vi "Example_Port Code_cRIO.vi"(10 "Port":u8, 11 "FPGA I/O":T1={"SCLK"="DIO15", "CS_1"="DIO13", "MOSI"="DIO14", "MISO"="DIO12", "CS_2"="DIO11"}) -> ()   [LabVIEW 2011]
uses:
  Controls/FPGA SPI_Port Loop State.ctl
  <vilib>/rvi/DataTransferAndStorage/Container/Common/niFpgaContainerState.ctl
  <vilib>/rvi/DataTransferAndStorage/Container/Common/niFpgaDataTypeControl.ctl
  <vilib>/rvi/DataTransferAndStorage/Container/Common/niFpgaContainerImplementationControl.ctl
  <vilib>/rvi/DataTransferAndStorage/Container/Common/niFpgaContainerArbitrationOptionsControl.ctl
  <vilib>/rvi/DataTransferAndStorage/Container/Common/niFpgaTransferTypeControl.ctl
  <vilib>/rvi/DataTransferAndStorage/Container/Common/niFpgaContainerInitializationParameters.ctl
  <vilib>/rvi/Memory/Memory_Types/niFpgaMemoryInterfaceConfiguration.ctl
  <vilib>/rvi/FIFO/Fifo_Types/niFpgaFifoControlLogicControl.ctl
  <vilib>/rvi/DataTransferAndStorage/Container/Common/niFpgaContainerMetaDataKey.ctl
  Controls/FPGA SPI_SPI Loop State.ctl
  <vilib>/Platform/TimedLoop/XDataNode/timing_clust.ctl
  <vilib>/Platform/TimedLoop/XDataNode/nitl_modes.ctl
  <vilib>/Platform/TimedLoop/XDataNode/wakeup.ctl
  <vilib>/rvi/DataTransferAndStorage/Container/Common/niFpgaContainerGetUniqueNameForEmu.vi
  <vilib>/rvi/DataTransferAndStorage/Container/Common/niFpgaContainerSetEmuInfo.vi
  <vilib>/rvi/eio/common/nirviEmuReportErrorAndStop.vi
  Code/FPGA SPI_Globals.vi
  <vilib>/rvi/FIFO/Fifo_Resource/nirvififoEmulationSetSize.vi
  <vilib>/rvi/eio/common/nirviEmuTemplateMethod_errors.vi
  <vilib>/rvi/LocalResourceManager/LocalResourceManager.xnode
  <vilib>/Platform/TimedLoop/XDataNode/XDataNode.xnode
  <vilib>/rvi/DataTransferAndStorage/Container/XNode/niFpgaContainer.xnode
  <vilib>/rvi/FIFO/Fifo_Resource/nirvififoEmulationRead.vi
  <vilib>/rvi/FIFO/Fifo_Resource/nirvififoEmulationWrite.vi
  <vilib>/eio/EIONode/EIONode.xnode
  <vilib>/Platform/TimedLoop/XDataNode/XDNodeRunTimeDep.lvlib
panel:
  # "12 and 11 are NC"
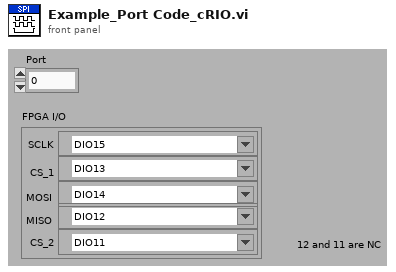
[diagram p1: front panel]
types:
  T1 = cluster{"SCLK":refnum<k21>, "CS_1":refnum<k21>, "MOSI":refnum<k21>, "MISO":refnum<k21>, "CS_2":refnum<k21>}
  T2 = cluster{"CS":u8, "CS Active State":bool, "CPOL":bool, "CPHA":bool, "Wait Ticks":u32}
  T3 = typedef "FPGA SPI_Port Loop State.ctl" = enum8{"Idle", "Start", "Configure Hardware", "Start Hardware", "Set Done", "Wait Until Done"}
  T4 = typedef "FPGA SPI_SPI Loop State.ctl" = enum8{"Initialize", "Read From FIFO", "Set CS", "Wait Before Set", "Set Clock", "Wait Before Reset", "Reset Clock", "Write to FIFO", "Reset CS"}
  T5 = typedef "XDNodeRunTimeDep.lvlib/timing_clust.ctl" = cluster{"Expected End [f-1]":u64, "Actual End [f-1]":u64, "Finished Late? [f-1]":bool, "Expected End [i-1]":u64, "Actual End [i-1]":u64, "Finished Late? [i-1]":bool, "Expected Start [i]":u64, "Actual Start [i]":u64, "Expected Start [f]":u64, "Actual Start [f]":u64, "Source Name":string, "Structure Name":string, "Period":i64, "Deadline":i64, "Offset":i64, "Start":i64, "Priority":i32, "Timeout":i32, "Mode":T6, "Wakeup Reason":T7, "Error":errorcluster, "Source Type":string, "Secondary Source Type":string, "Global End Time":u64, "Global Start Time":u64, "Frame Duration":u64, "Iteration Duration":u64, "Assigned CPU":i32, "I/O Scan Engine Mode":u32}
  T6 = typedef "XDNodeRunTimeDep.lvlib/nitl_modes.ctl" = enum32{"No Change", "Process missed periods, maintain original phase", "Discard missed periods, maintain original phase", "Process missed periods, ignore original phase", "Discard missed periods, ignore original phase"}
  T7 = typedef "XDNodeRunTimeDep.lvlib/wakeup.ctl" = enum32{"Normal", "Aborted", "Asynchronous wakeup", "Timing source error", "Timed loop error", "Timeout"}
  T8 = typedef "FPGA SPI_Cmd.ctl" = enum8{"Idle", "Write/Read SPI", "Configure"}
  T9 = cluster{"MOSI":bool[], "MISO":bool[], "MOSI Byte Index":i8, "MISO Byte Index":i8}
  T10 = cluster{"Next State":T4, "Wait Count":u32, "Total Bits":u16, "Current Bit":u16, "Total Bytes":u16}
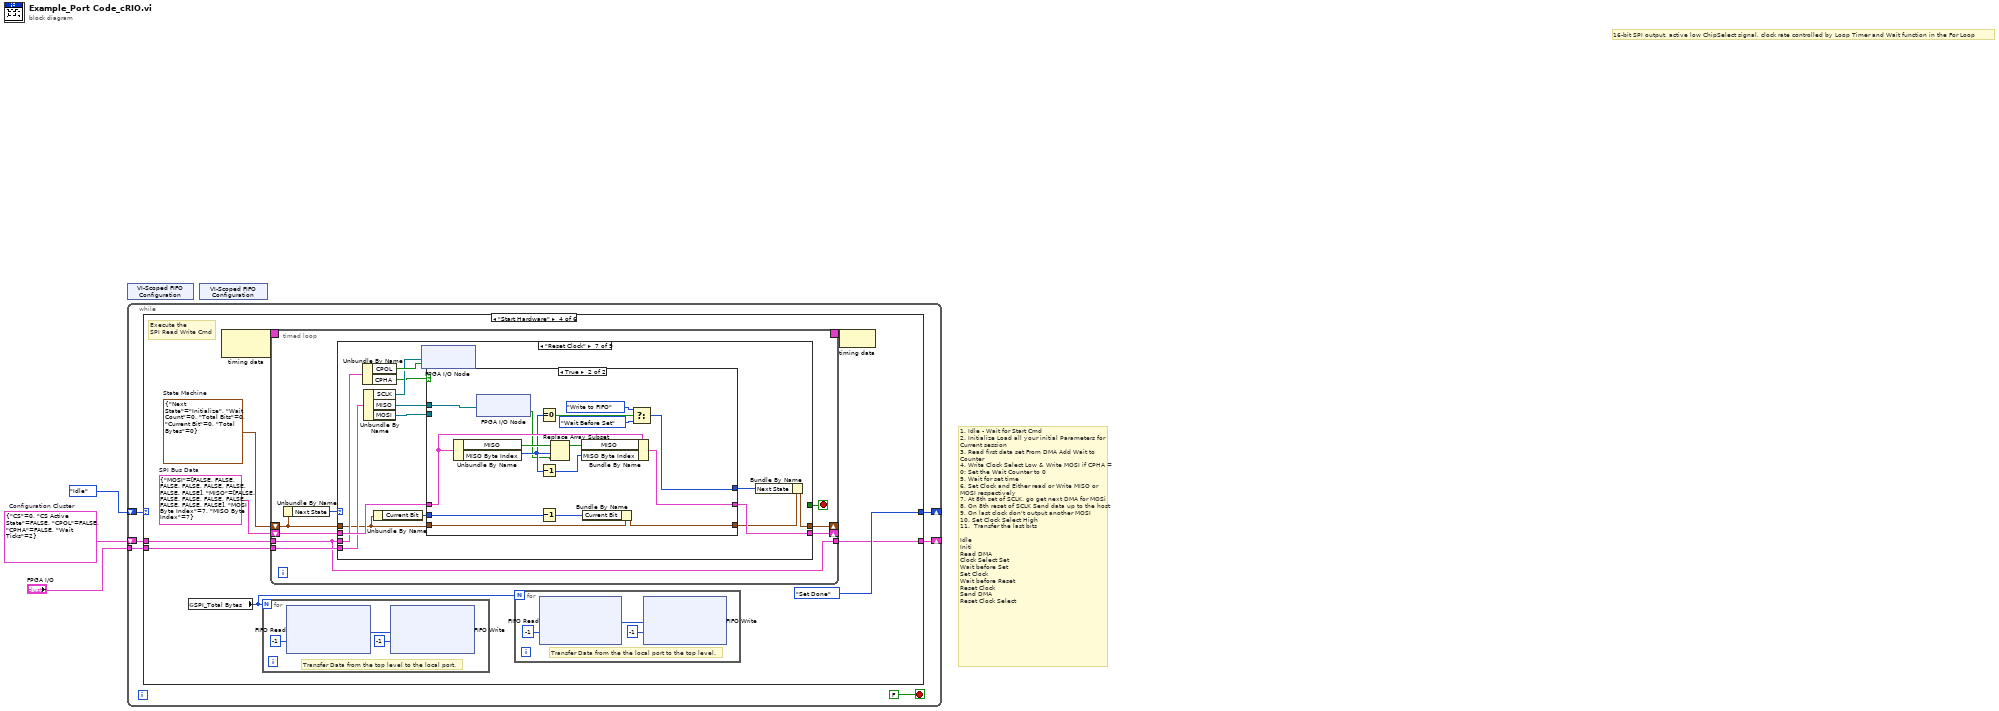
[diagram p0: block diagram]
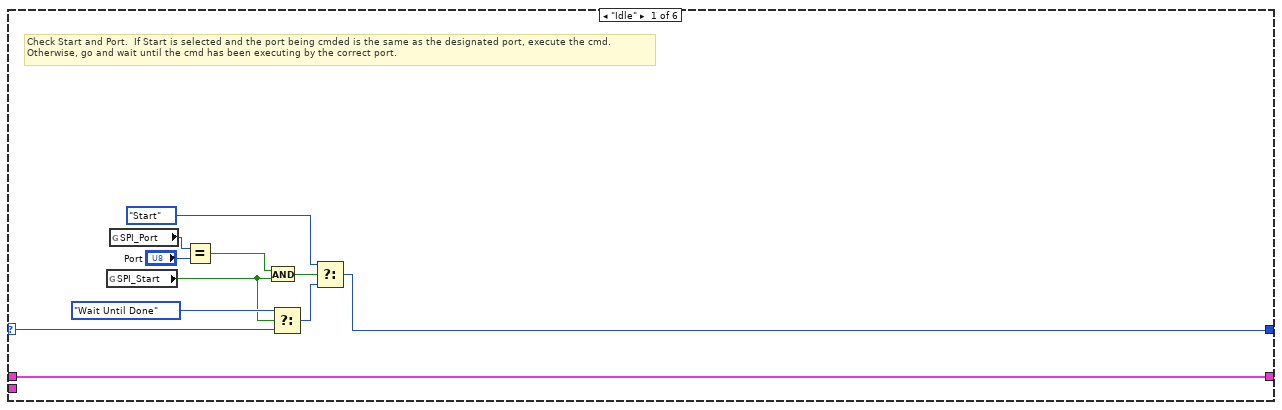
[diagram p2: hidden frame]
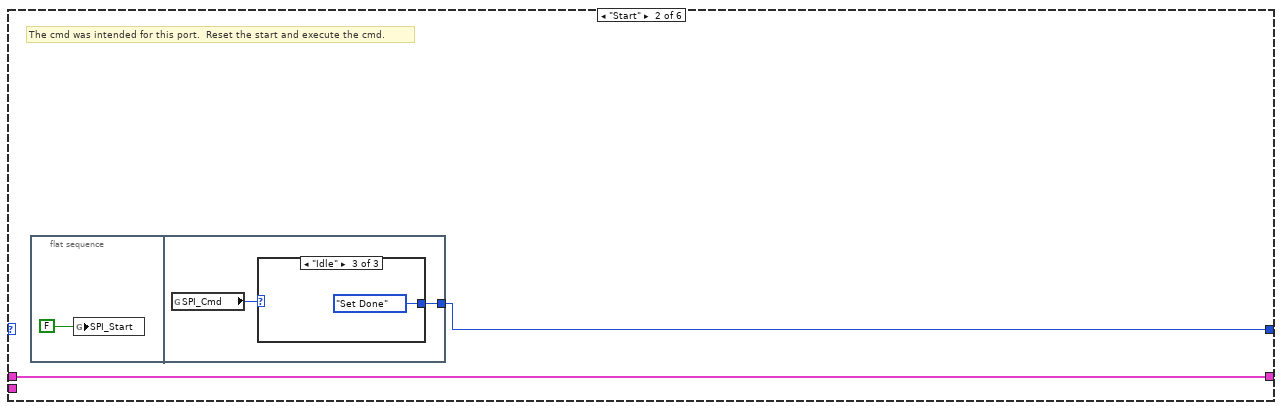
[diagram p3: hidden frame]
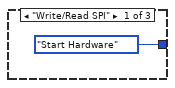
[diagram p4: hidden frame]
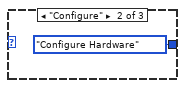
[diagram p5: hidden frame]
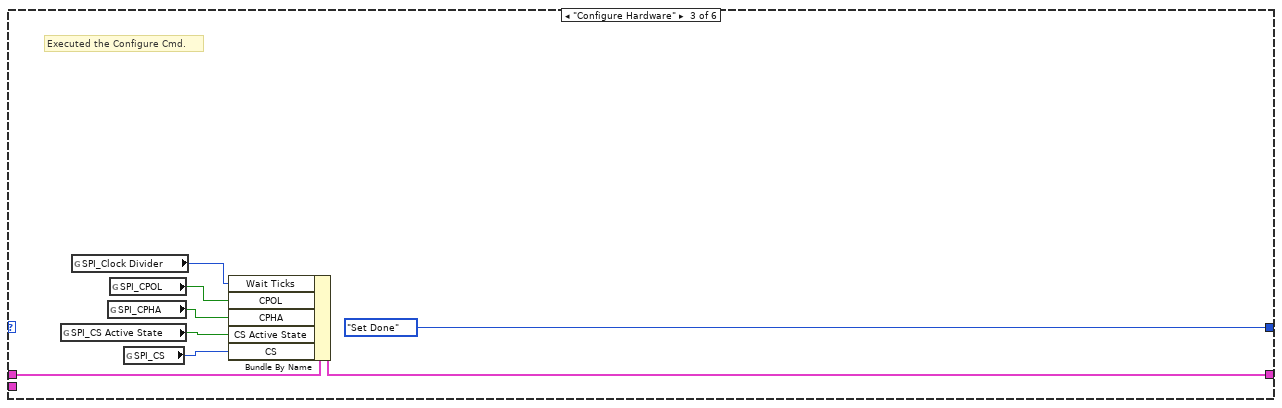
[diagram p6: hidden frame]
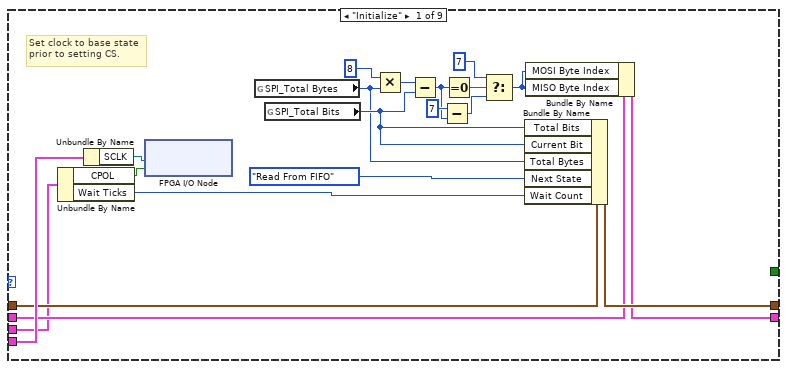
[diagram p7: hidden frame]
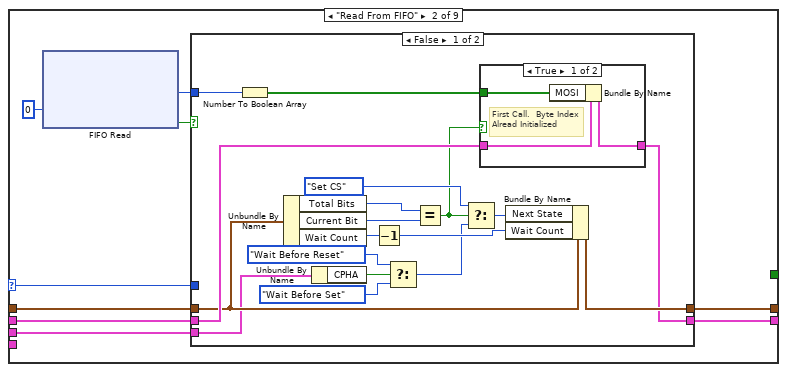
[diagram p8: hidden frame]
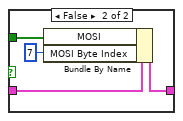
[diagram p9: hidden frame]
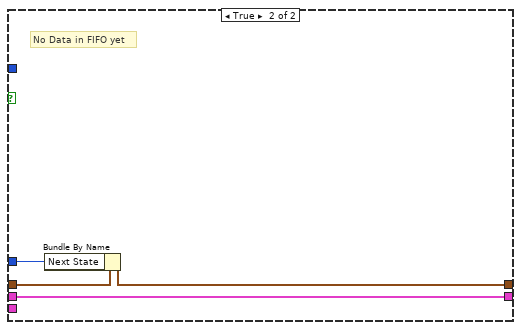
[diagram p10: hidden frame]
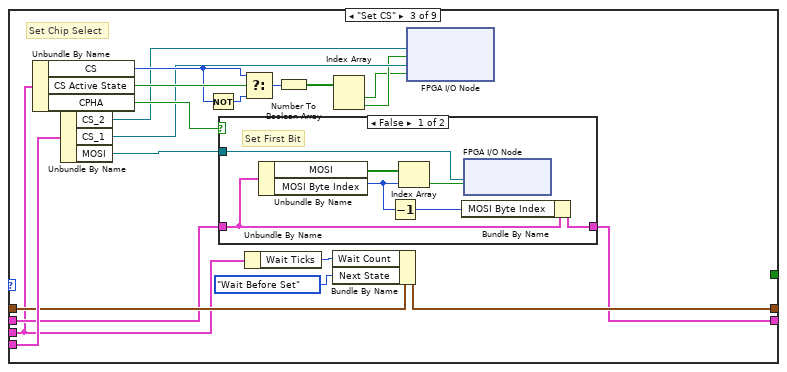
[diagram p11: hidden frame]
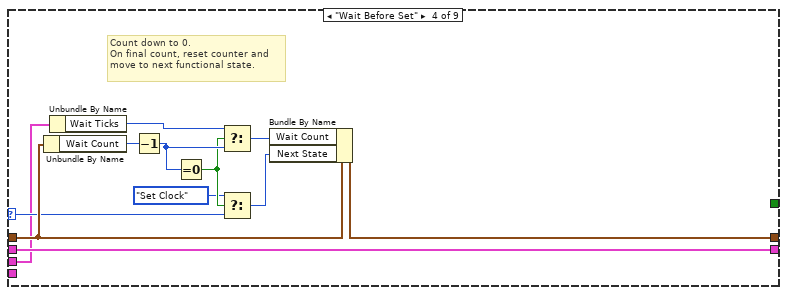
[diagram p13: hidden frame]
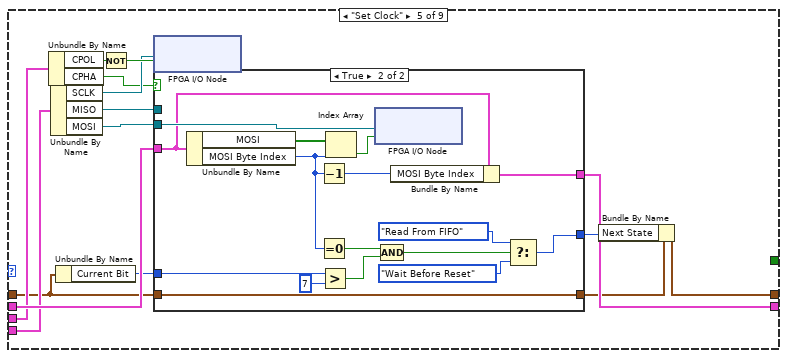
[diagram p14: hidden frame]
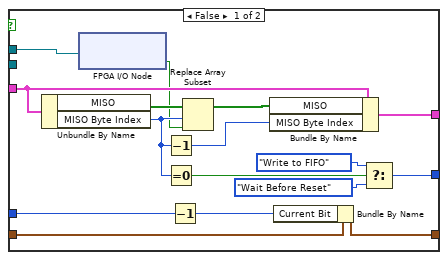
[diagram p15: hidden frame]
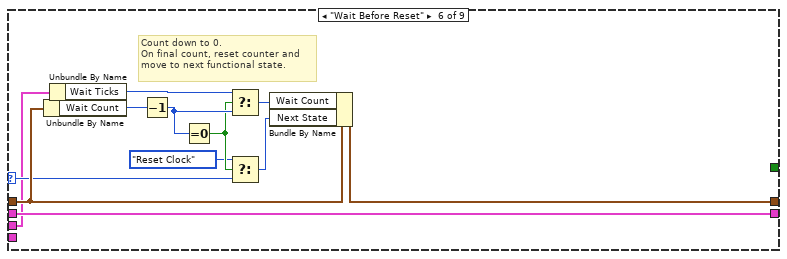
[diagram p16: hidden frame]
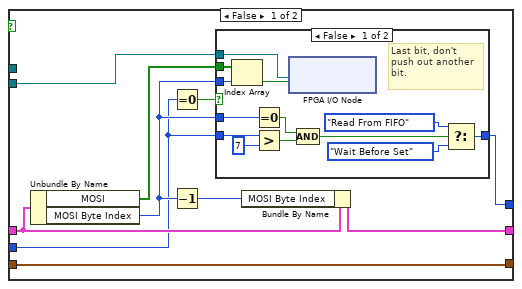
[diagram p17: hidden frame]
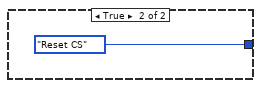
[diagram p18: hidden frame]
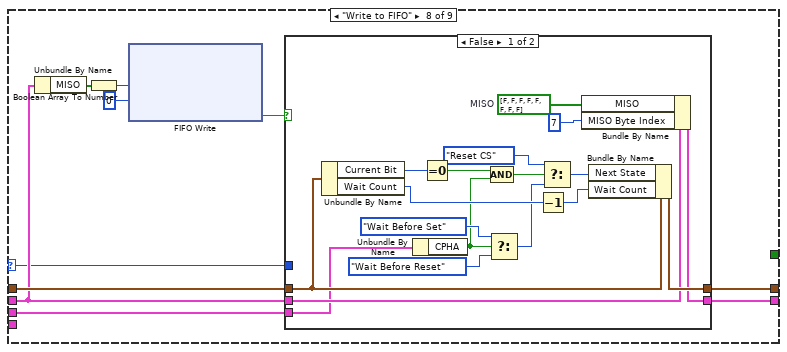
[diagram p19: hidden frame]
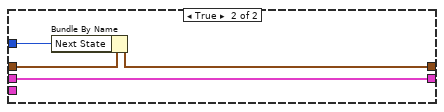
[diagram p20: hidden frame]
diagram:
  w2 = T2 {"CS"=0, "CS Active State"=FALSE, "CPOL"=FALSE, "CPHA"=FALSE, "Wait Ticks"=2}  # Configuration Cluster
  # "16-bit SPI output, active low ChipSelect signal, clock rate controlled by Loop Timer and Wait function in the For Loop"
  # "1. Idle - Wait for Start Cmd\n2. Initialize Load all your initial Parameters for Current session\n3. Read first data set From DMA Add Wait to Counter\n4. Write Clock Select Low & Write MOSI if CPHA = 0; Set the Wait Counter to 0\n5. Wait for set time\n6. Set Clock and Either read or Write MISO or MOSI respectively\n7. At 8th set of SCLK, go get next DMA for MOSi\n8. On 8th reset of SCLK Send data up to the host\n9. On last clock don't output another MOSI\n10. Set Clock Select High \n11.  Transfer the last bits\n\nIdle\nIniti\nRead DMA\nClock Select Set\nWait before Set\nSet Clock\nWait before Reset\nReset Clock\nSend DMA\nReset Clock Select"
  n1 = xnode "VI-Scoped FIFO Configuration"() -> ()  [unwired: 1 out]
  n2 = while {
    shift-right: [w8] -> _
    shift-left: FPGA_SPI_Port_Loop_State."Idle" ("Action") -> [w7]
    shift-right: [w4] -> _
    shift-left: w2 -> [w6]
    tunnel: "FPGA I/O" -> [w5]
    stop <- FALSE stop-if-true
    n3 = case shown="\"Start Hardware\"" w7 {
      selector: w7 -> [w10 _ _ _ _ w322]
      tunnel: [w19 w22 FPGA_SPI_Port_Loop_State."Set Done" ("Action") FPGA_SPI_Port_Loop_State."Set Done" ("Action") FPGA_SPI_Port_Loop_State."Idle" ("Action") w321] -> w8
      tunnel: w6 -> [w14 w21 w32 w37 w317 w320]
      tunnel: w5 -> [_ _ _ w42 _ _]
      tunnel: [w14 w21 w31 w38 w317 w320] -> w4
      frame "Idle" {
        # "Check Start and Port.  If Start is selected and the port being cmded is the same as the designated port, execute the cmd.\nOtherwise, go and wait until the cmd has been executing by the correct port."
        n4 = global read "FPGA SPI_Globals.vi" "SPI_Start"() -> (w11:bool)
        n5 = global read "FPGA SPI_Globals.vi" "SPI_Port"() -> (w18:u8)
        n6 = Equal?(x=w18, y="Port") -> (x = y?=w12:bool)
        n7 = And(x=w12, y=w11) -> (x .and. y?=w16:bool)
        n8 = Select(t=FPGA_SPI_Port_Loop_State."Wait Until Done" ("Action"), s=w11, f=w10) -> (s? t:f=w15:T3)
        n9 = Select(t=FPGA_SPI_Port_Loop_State."Start" ("Action"), s=w16, f=w15) -> (s? t:f=w19:T3)
      }
      frame "Start" {
        # "The cmd was intended for this port.  Reset the start and execute the cmd."
        n10 = flat-sequence {
          tunnel: [w24] -> w22
          frame #0 {
            n11 = global write "FPGA SPI_Globals.vi" "SPI_Start"(FALSE ("Write Flag")) -> ()
          }
          frame #1 {
            n12 = global read "FPGA SPI_Globals.vi" "SPI_Cmd"() -> (w25:T8)
            n13 = case shown="\"Idle\"" w25 {
              tunnel: [FPGA_SPI_Port_Loop_State."Start Hardware" ("Action") FPGA_SPI_Port_Loop_State."Configure Hardware" ("Action") FPGA_SPI_Port_Loop_State."Set Done" ("Action")] -> w24
              frame "Write/Read SPI" {
              }
              frame "Configure" {
              }
              frame "Idle" {
              }
            }
          }
        }
      }
      frame "Configure Hardware" {
        # "Executed the Configure Cmd."
        n14 = global read "FPGA SPI_Globals.vi" "SPI_CS Active State"() -> (w34:bool)
        n15 = global read "FPGA SPI_Globals.vi" "SPI_Clock Divider"() -> (w29:u32)
        n16 = global read "FPGA SPI_Globals.vi" "SPI_CPHA"() -> (w33:bool)
        n17 = global read "FPGA SPI_Globals.vi" "SPI_CPOL"() -> (w36:bool)
        n18 = global read "FPGA SPI_Globals.vi" "SPI_CS"() -> (w35:u8)
        n19 = Bundle By Name(cluster=w32, "Wait Ticks"=w29, "CPOL"=w36, "CPHA"=w33, "CS Active State"=w34, "CS"=w35) -> (w31:T2)
      }
      frame "Start Hardware" {
        w40 = T9 {"MOSI"=[FALSE, FALSE, FALSE, FALSE, FALSE, FALSE, FALSE, FALSE], "MISO"=[FALSE, FALSE, FALSE, FALSE, FALSE, FALSE, FALSE, FALSE], "MOSI Byte Index"=7, "MISO Byte Index"=7}  # SPI Bus Data
        w41 = T10 {"Next State"=enum."Initialize", "Wait Count"=0, "Total Bits"=0, "Current Bit"=0, "Total Bytes"=0}  # State Machine
        # "Execute the \nSPI Read Write Cmd"
        n20 = global read "FPGA SPI_Globals.vi" "SPI_Total Bytes"() -> (w39:u16)
        n21 = node-c288() -> (w44:T5)  [unwired: 1 out]
        n22 = for {
          N: w39 -> [_]
          # "Transfer Data from the top level to the local port."
          n23 = xnode ("FIFO Read")("Timeout"=-1) -> ("Element"=w50:u8)  [unwired: 1 in, 2 out]
          n24 = xnode ("FIFO Write")("Element"=w50, "Timeout"=-1) -> ()  [unwired: 1 in, 2 out]
        }
        n25 = timed-loop {
          timing-out: [_] -> w43
          timing: w44 -> [_]
          shift-right: [w59] -> _
          shift-left: w41 -> [w58]
          shift-right: [w55] -> _
          shift-left: w40 -> [w56]
          tunnel: w42 -> [w53]
          tunnel: [w52] -> w38
          tunnel: w37 -> [w52]
          stop <- w54 stop-if-true
          n26 = Unbundle By Name(w58) -> ("Next State"=w57:T4)
          n27 = case shown="\"Reset Clock\"" w57 {
            selector: w57 -> [_ w80 _ w149 _ w207 _ w270 _]
            tunnel: w58 -> [w76 w83 w129 w155 w159 w214 w217 w276 w311]
            tunnel: [w75 w86 w136 w156 w171 w215 w229 w277 w312] -> w59
            tunnel: w52 -> [w61 w82 w124 w146 w166 w205 w225 w274 w308]
            tunnel: w56 -> [w62 w84 w126 w147 w167 w212 w227 w273 w309]
            tunnel: [w65 w85 w125 w147 w168 w212 w226 w272 w309] -> w55
            tunnel: w53 -> [w79 _ w133 _ w165 _ w224 _ w306]
            tunnel: [_ _ _ _ _ _ _ _ TRUE ("Start Hardware")] -> w54
            frame "Initialize" {
              # "Set clock to base state\nprior to setting CS."
              n28 = Unbundle By Name(w61) -> ("CPOL"=w77:bool, "Wait Ticks"=w60:u32)
              n29 = Unbundle By Name(w79) -> ("SCLK"=w78:refnum<k21>)
              n30 = xnode "FPGA I/O Node"("I/O Item"=w77, "FPGA I/O In"=w78) -> ()  [unwired: 1 out]
              n31 = global read "FPGA SPI_Globals.vi" "SPI_Total Bytes"() -> (w63:u16)
              n32 = global read "FPGA SPI_Globals.vi" "SPI_Total Bits"() -> (w64:u16)
              n33 = Multiply(x=u16 8 ("y"), y=w63) -> (x*y=w72:u16)
              n34 = Subtract(x=w72, y=w64) -> (x-y=w69:i8)
              n35 = Subtract(x=i8 7, y=w69) -> (x-y=w67:i8)
              n36 = Equal To 0?(x=w69) -> (x = 0?=w68:bool)
              n37 = Select(t=i8 7 ("y"), s=w68, f=w67) -> (s? t:f=w66:i8)
              n38 = Bundle By Name(cluster=w76, "Total Bits"=w64, "Current Bit"=w64, "Total Bytes"=w63, "Next State"=FPGA_SPI_SPI_Loop_State."Read From FIFO", "Wait Count"=w60) -> (w75:T10)
              n39 = Bundle By Name(cluster=w62, "MOSI Byte Index"=w66, "MISO Byte Index"=w66) -> (w65:T9)
            }
            frame "Read From FIFO" {
              n40 = xnode ("FIFO Read")("Timeout"=0) -> ("Element"=w87:u8, "Timed Out?"=w81:bool)  [unwired: 1 in, 1 out]
              n41 = case shown="False" w81 {
                tunnel: w87 -> [w106 _]
                tunnel: [w105 w114] -> w86
                tunnel: [w100 w117] -> w85
                tunnel: w84 -> [w99 w117]
                tunnel: w83 -> [w97 w115]
                tunnel: w82 -> [w89 _]
                tunnel: w80 -> [_ w116]
                frame False {
                  n42 = Number To Boolean Array(number=w106) -> (Boolean array=w98:bool[])
                  n43 = Unbundle By Name(w97) -> ("Total Bits"=w102:u16, "Current Bit"=w104:u16, "Wait Count"=w96:u32)
                  n44 = Unbundle By Name(w89) -> ("CPHA"=w93:bool)
                  n45 = Decrement(x=w96) -> (x-1=w95:u32)
                  n46 = Select(t=FPGA_SPI_SPI_Loop_State."Wait Before Reset" ("Next State"), s=w93, f=FPGA_SPI_SPI_Loop_State."Wait Before Set" ("Next State")) -> (s? t:f=w90:T4)
                  n47 = Equal?(x=w102, y=w104) -> (x = y?=w94:bool)
                  n48 = Select(t=FPGA_SPI_SPI_Loop_State."Set CS" ("Next State"), s=w94, f=w90) -> (s? t:f=w101:T4)
                  n49 = case shown="True" w94 {
                    tunnel: [w109 w113] -> w100
                    tunnel: w99 -> [w108 w112]
                    tunnel: w98 -> [w107 w111]
                    frame True {
                      # "First Call.  Byte Index Alread Initialized"
                      n50 = Bundle By Name(cluster=w108, "MOSI"=w107) -> (w109:T9)
                    }
                    frame False {
                      n51 = Bundle By Name(cluster=w112, "MOSI"=w111, "MOSI Byte Index"=i8 7) -> (w113:T9)
                    }
                  }
                  n52 = Bundle By Name(cluster=w97, "Next State"=w101, "Wait Count"=w95) -> (w105:T10)
                }
                frame True {
                  # "No Data in FIFO yet"
                  n53 = Bundle By Name(cluster=w115, "Next State"=w116) -> (w114:T10)
                }
              }
            }
            frame "Set CS" {
              # "Set Chip Select"
              n54 = Unbundle By Name(w124) -> ("CS"=w130:u8, "CS Active State"=w135:bool, "CPHA"=w131:bool)
              n55 = Unbundle By Name(w133) -> ("CS_2"=w118:refnum<k21>, "CS_1"=w122:refnum<k21>, "MOSI"=w132:refnum<k21>)
              n56 = Not(x=w130) -> (.not. x?=w134:u8)
              n57 = case shown="False" w131 {
                tunnel: w126 -> [w140 w144]
                tunnel: w132 -> [w142 _]
                tunnel: [w138 w144] -> w125
                frame False {
                  # "Set First Bit"
                  n58 = Unbundle By Name(w140) -> ("MOSI"=w143:bool[], "MOSI Byte Index"=w141:i8)
                  n59 = Decrement(x=w141) -> (x-1=w139:i8)
                  n60 = Index Array(array=w143, index=w141) -> (element=w137:bool)
                  n61 = Bundle By Name(cluster=w140, "MOSI Byte Index"=w139) -> (w138:T9)
                  n62 = xnode "FPGA I/O Node"("I/O Item"=w137, "FPGA I/O In"=w142) -> ()  [unwired: 1 out]
                }
                frame True {
                }
              }
              n63 = Select(t=w130, s=w135, f=w134) -> (s? t:f=w123:u8)
              n64 = Unbundle By Name(w124) -> ("Wait Ticks"=w128:u32)
              n65 = Number To Boolean Array(number=w123) -> (Boolean array=w121:bool[])
              n66 = Bundle By Name(cluster=w129, "Wait Count"=w128, "Next State"=FPGA_SPI_SPI_Loop_State."Wait Before Set" ("Enum")) -> (w136:T10)
              n67 = Index Array(array=w121) -> (element #1=w119:bool, element #2=w120:bool)  [unwired: 2 in]
              n68 = xnode "FPGA I/O Node"("I/O Item"=w120, "FPGA I/O In"=w118, "I/O Item"=w119, "FPGA I/O In"=w122) -> ()  [unwired: 2 out]
            }
            frame "Wait Before Set" {
              # "Count down to 0.\nOn final count, reset counter and\nmove to next functional state."
              n69 = Unbundle By Name(w155) -> ("Wait Count"=w153:u32)
              n70 = Unbundle By Name(w146) -> ("Wait Ticks"=w145:u32)
              n71 = Decrement(x=w153) -> (x-1=w154:u32)
              n72 = Equal To 0?(x=w154) -> (x = 0?=w152:bool)
              n73 = Select(t=w145, s=w152, f=w154) -> (s? t:f=w151:u32)
              n74 = Select(t=FPGA_SPI_SPI_Loop_State."Set Clock", s=w152, f=w149) -> (s? t:f=w150:T4)
              n75 = Bundle By Name(cluster=w155, "Wait Count"=w151, "Next State"=w150) -> (w156:T10)
            }
            frame "Set Clock" {
              n76 = Unbundle By Name(w166) -> ("CPOL"=w169:bool, "CPHA"=w161:bool)
              n77 = Unbundle By Name(w165) -> ("SCLK"=w162:refnum<k21>, "MISO"=w163:refnum<k21>, "MOSI"=w164:refnum<k21>)
              n78 = Unbundle By Name(w159) -> ("Current Bit"=w158:u16)
              n79 = Not(x=w169) -> (.not. x?=w170:bool)
              n80 = xnode "FPGA I/O Node"("I/O Item"=w170, "FPGA I/O In"=w162) -> ()  [unwired: 1 out]
              n81 = case shown="True" w161 {
                tunnel: [w187 w191] -> w168
                tunnel: w167 -> [w186 w192]
                tunnel: w164 -> [_ w202]
                tunnel: w163 -> [w182 _]
                tunnel: w159 -> [w181 w201]
                tunnel: [w180 w201] -> w160
                tunnel: w158 -> [w179 w199]
                tunnel: [w174 w193] -> w157
                frame False {
                  n82 = Unbundle By Name(w186) -> ("MISO"=w185:bool[], "MISO Byte Index"=w178:i8)
                  n83 = xnode "FPGA I/O Node"("FPGA I/O In"=w182) -> ("I/O Item"=w172:bool)  [unwired: 1 out]
                  n84 = Decrement(x=w178) -> (x-1=w183:i8)
                  n85 = Equal To 0?(x=w178) -> (x = 0?=w173:bool)
                  n86 = Decrement(x=w179) -> (x-1=w177:u16)
                  n87 = Replace Array Subset(array=w185, new element=w172, index=w178) -> (w184:bool[])
                  n88 = Bundle By Name(cluster=w186, "MISO"=w184, "MISO Byte Index"=w183) -> (w187:T9)
                  n89 = Bundle By Name(cluster=w181, "Current Bit"=w177) -> (w180:T10)
                  n90 = Select(t=FPGA_SPI_SPI_Loop_State."Write to FIFO" ("Enum"), s=w173, f=FPGA_SPI_SPI_Loop_State."Wait Before Reset" ("Enum")) -> (s? t:f=w174:T4)
                }
                frame True {
                  n91 = Unbundle By Name(w192) -> ("MOSI"=w203:bool[], "MOSI Byte Index"=w190:i8)
                  n92 = Decrement(x=w190) -> (x-1=w189:i8)
                  n93 = Equal To 0?(x=w190) -> (x = 0?=w200:bool)
                  n94 = Greater?(x=w199, y=u16 7 ("x")) -> (0:w197:bool)
                  n95 = Index Array(array=w203, index=w190) -> (element=w188:bool)
                  n96 = xnode "FPGA I/O Node"("I/O Item"=w188, "FPGA I/O In"=w202) -> ()  [unwired: 1 out]
                  n97 = Compound Arithmetic op=AND(w200, w197) -> (w196:bool)
                  n98 = Bundle By Name(cluster=w192, "MOSI Byte Index"=w189) -> (w191:T9)
                  n99 = Select(t=FPGA_SPI_SPI_Loop_State."Read From FIFO" ("Enum"), s=w196, f=FPGA_SPI_SPI_Loop_State."Wait Before Reset" ("Enum")) -> (s? t:f=w193:T4)
                }
              }
              n100 = Bundle By Name(cluster=w160, "Next State"=w157) -> (w171:T10)
            }
            frame "Wait Before Reset" {
              # "Count down to 0.\nOn final count, reset counter and\nmove to next functional state."
              n101 = Unbundle By Name(w214) -> ("Wait Count"=w211:u32)
              n102 = Unbundle By Name(w205) -> ("Wait Ticks"=w204:u32)
              n103 = Decrement(x=w211) -> (x-1=w213:u32)
              n104 = Equal To 0?(x=w213) -> (x = 0?=w210:bool)
              n105 = Select(t=w204, s=w210, f=w213) -> (s? t:f=w209:u32)
              n106 = Select(t=FPGA_SPI_SPI_Loop_State."Reset Clock", s=w210, f=w207) -> (s? t:f=w208:T4)
              n107 = Bundle By Name(cluster=w214, "Wait Count"=w209, "Next State"=w208) -> (w215:T10)
            }
            frame "Reset Clock" {
              n108 = Unbundle By Name(w225) -> ("CPOL"=w228:bool, "CPHA"=w220:bool)
              n109 = Unbundle By Name(w224) -> ("SCLK"=w221:refnum<k21>, "MISO"=w222:refnum<k21>, "MOSI"=w223:refnum<k21>)
              n110 = Unbundle By Name(w217) -> ("Current Bit"=w216:u16)
              n111 = xnode "FPGA I/O Node"("I/O Item"=w228, "FPGA I/O In"=w221) -> ()  [unwired: 1 out]
              n112 = case shown="True" w220 {
                tunnel: [w234 w266] -> w226
                tunnel: w227 -> [w235 w269]
                tunnel: w223 -> [w239 _]
                tunnel: w222 -> [_ w267]
                tunnel: w217 -> [w236 w264]
                tunnel: [w236 w263] -> w219
                tunnel: [w230 w257] -> w218
                tunnel: w216 -> [w231 w255]
                frame False {
                  n113 = Unbundle By Name(w235) -> ("MOSI"=w238:bool[], "MOSI Byte Index"=w232:i8)
                  n114 = Equal To 0?(x=w231) -> (x = 0?=w237:bool)
                  n115 = Decrement(x=w232) -> (x-1=w233:i8)
                  n116 = case shown="False" w237 {
                    tunnel: w239 -> [w252 _]
                    tunnel: w238 -> [w251 _]
                    tunnel: w232 -> [w250 _]
                    tunnel: w232 -> [w246 _]
                    tunnel: w231 -> [w245 _]
                    tunnel: [w241 FPGA_SPI_SPI_Loop_State."Reset CS" ("Enum")] -> w230
                    frame False {
                      # "Last bit, don't\npush out another\nbit."
                      n117 = Index Array(array=w251, index=w250) -> (element=w240:bool)
                      n118 = Equal To 0?(x=w246) -> (x = 0?=w248:bool)
                      n119 = Greater?(x=w245, y=u16 7 ("x")) -> (0:w249:bool)
                      n120 = xnode "FPGA I/O Node"("I/O Item"=w240, "FPGA I/O In"=w252) -> ()  [unwired: 1 out]
                      n121 = Compound Arithmetic op=AND(w248, w249) -> (w242:bool)
                      n122 = Select(t=FPGA_SPI_SPI_Loop_State."Read From FIFO" ("Enum"), s=w242, f=FPGA_SPI_SPI_Loop_State."Wait Before Set" ("Enum")) -> (s? t:f=w241:T4)
                    }
                    frame True {
                    }
                  }
                  n123 = Bundle By Name(cluster=w235, "MOSI Byte Index"=w233) -> (w234:T9)
                }
                frame True {
                  n124 = Unbundle By Name(w269) -> ("MISO"=w268:bool[], "MISO Byte Index"=w259:i8)
                  n125 = xnode "FPGA I/O Node"("FPGA I/O In"=w267) -> ("I/O Item"=w254:bool)  [unwired: 1 out]
                  n126 = Equal To 0?(x=w259) -> (x = 0?=w256:bool)
                  n127 = Decrement(x=w259) -> (x-1=w262:i8)
                  n128 = Decrement(x=w255) -> (x-1=w258:u16)
                  n129 = Replace Array Subset(array=w268, new element=w254, index=w259) -> (w265:bool[])
                  n130 = Bundle By Name(cluster=w269, "MISO"=w265, "MISO Byte Index"=w262) -> (w266:T9)
                  n131 = Bundle By Name(cluster=w264, "Current Bit"=w258) -> (w263:T10)
                  n132 = Select(t=FPGA_SPI_SPI_Loop_State."Write to FIFO" ("Enum"), s=w256, f=FPGA_SPI_SPI_Loop_State."Wait Before Set" ("Enum")) -> (s? t:f=w257:T4)
                }
              }
              n133 = Bundle By Name(cluster=w219, "Next State"=w218) -> (w229:T10)
            }
            frame "Write to FIFO" {
              n134 = Unbundle By Name(w273) -> ("MISO"=w279:bool[])
              n135 = Boolean Array To Number(Boolean array=w279) -> (number=w278:u8)
              n136 = xnode ("FIFO Write")("Element"=w278, "Timeout"=0) -> ("Timed Out?"=w271:bool)  [unwired: 1 in, 1 out]
              n137 = case shown="False" w271 {
                tunnel: [w297 w299] -> w277
                tunnel: w276 -> [w296 w300]
                tunnel: w274 -> [w280 _]
                tunnel: w273 -> [w283 w301]
                tunnel: [w281 w301] -> w272
                tunnel: w270 -> [_ w298]
                frame False {
                  w284 = bool[] [FALSE, FALSE, FALSE, FALSE, FALSE, FALSE, FALSE, FALSE]  # MISO
                  n138 = Unbundle By Name(w296) -> ("Current Bit"=w295:u16, "Wait Count"=w292:u32)
                  n139 = Unbundle By Name(w280) -> ("CPHA"=w286:bool)
                  n140 = Equal To 0?(x=w295) -> (x = 0?=w288:bool)
                  n141 = Select(t=FPGA_SPI_SPI_Loop_State."Wait Before Set" ("Next State"), s=w286, f=FPGA_SPI_SPI_Loop_State."Wait Before Reset" ("Next State")) -> (s? t:f=w289:T4)
                  n142 = Compound Arithmetic op=AND(w288, w286) -> (w287:bool)
                  n143 = Decrement(x=w292) -> (x-1=w285:u32)
                  n144 = Select(t=FPGA_SPI_SPI_Loop_State."Reset CS" ("Next State"), s=w287, f=w289) -> (s? t:f=w293:T4)
                  n145 = Bundle By Name(cluster=w283, "MISO"=w284, "MISO Byte Index"=i8 7) -> (w281:T9)
                  n146 = Bundle By Name(cluster=w296, "Next State"=w293, "Wait Count"=w285) -> (w297:T10)
                }
                frame True {
                  n147 = Bundle By Name(cluster=w300, "Next State"=w298) -> (w299:T10)
                }
              }
            }
            frame "Reset CS" {
              # "Reset all CS signals.  Stop the loop."
              n148 = Unbundle By Name(w308) -> ("CS Active State"=w307:bool)
              n149 = Unbundle By Name(w306) -> ("CS_2"=w302:refnum<k21>, "CS_1"=w305:refnum<k21>)
              n150 = Not(x=w307) -> (.not. x?=w303:bool)
              n151 = Bundle By Name(cluster=w311, "Next State"=FPGA_SPI_SPI_Loop_State."Initialize" ("Enum")) -> (w312:T10)
              n152 = xnode "FPGA I/O Node"("I/O Item"=w303, "FPGA I/O In"=w302, "I/O Item"=w303, "FPGA I/O In"=w305) -> ()  [unwired: 2 out]
            }
          }
        }
        n153 = for {
          N: w39 -> [_]
          # "Transfer Data from the the local port to the top level."
          n154 = xnode ("FIFO Read")("Timeout"=-1) -> ("Element"=w47:u8)  [unwired: 1 in, 2 out]
          n155 = xnode ("FIFO Write")("Element"=w47, "Timeout"=-1) -> ()  [unwired: 1 in, 2 out]
        }
        n156 = node-c288(w43) -> ()
      }
      frame "Set Done" {
        # "Set the done flag"
        n157 = global write "FPGA SPI_Globals.vi" "SPI_Done"(TRUE ("Done")) -> ()
      }
      frame "Wait Until Done" {
        # "Wait until the executing port finishes."
        n158 = global read "FPGA SPI_Globals.vi" "SPI_Done"() -> (w324:bool)
        n159 = Select(t=FPGA_SPI_Port_Loop_State."Idle" ("Action"), s=w324, f=w322) -> (s? t:f=w321:T3)
      }
    }
  }
  n160 = xnode "VI-Scoped FIFO Configuration"() -> ()  [unwired: 1 out]
